vi "Write byte orders.vi"(8 "error in":errorcluster, 10 "byte orders":T1[](array[typedef]), 11 "Profibus Module configuration in":refnum<class "Profibus Module configuration.lvclass">) -> (0 "error out":errorcluster, 3 "Profibus Module configuration out":refnum<class "Profibus Module configuration.lvclass">)   [LabVIEW 2013, in "Profibus Module configuration.lvclass"]
uses:
  Profibus Module configuration.lvclass
  endianness setting.ctl
  Profibus Module configuration.lvclass/Profibus Module configuration.ctl
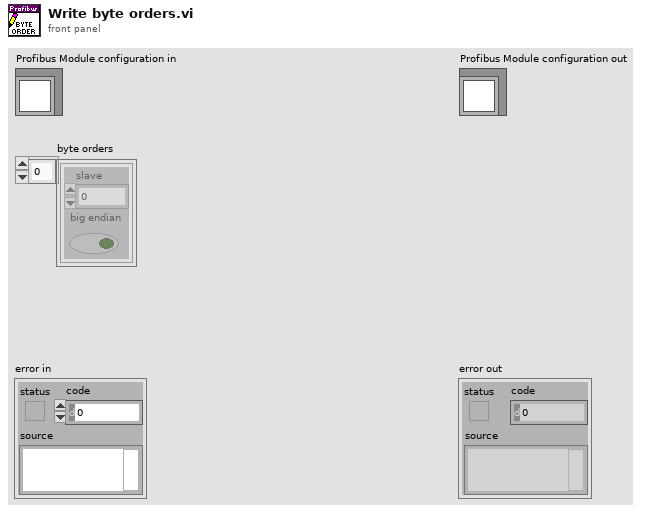
[diagram p1: front panel]
types:
  T1 = typedef "Profibus Module configuration.lvclass/endianness setting.ctl" = cluster{"slave":i8, "big endian":bool}
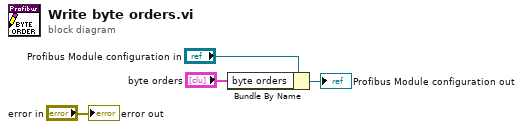
[diagram p0: block diagram]
diagram:
  n1 = Bundle By Name(cluster="Profibus Module configuration in", "byte orders"="byte orders") -> (→"Profibus Module configuration out":refnum<class "Profibus Module configuration.lvclass">)
  "error out" <- "error in"
